vi "Read Log File Directory.vi"(8 "error in (no error)":errorcluster, 11 "Check Size Message in":refnum<class "Check Size Message.lvclass">) -> (0 "error out":errorcluster, 2 "Log File Directory":string, 3 "Check Size Message out":refnum<class "Check Size Message.lvclass">)   [LabVIEW 2020, in "AIM ARINC 664 Engine.lvlib" / "Implementation.lvlib" / "Frame Logging.lvlib" / "Check Size Message.lvclass"]
uses:
  Check Size Message.lvclass
  Check Size Message.lvclass/Check Size Message.ctl
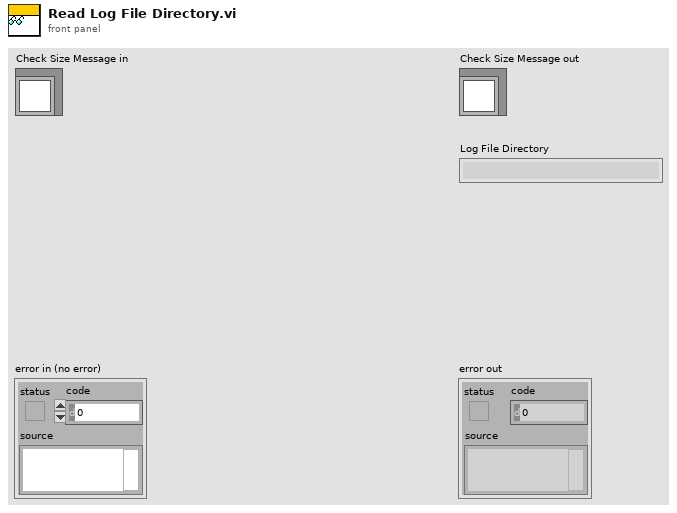
[diagram p1: front panel]
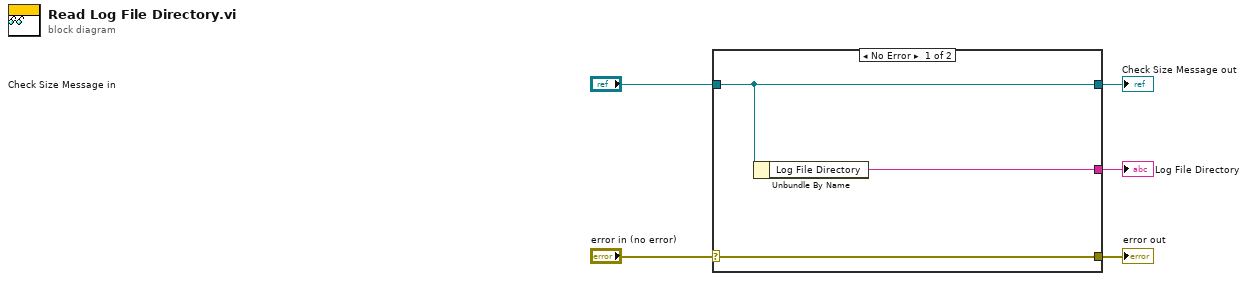
[diagram p0: block diagram]
diagram:
  n1 = case shown="No Error" "error in (no error)" {
    selector: "error in (no error)" -> [w8 w9]
    tunnel: [w8 w9] -> w4
    tunnel: [w7 w10] -> w2
    tunnel: "Check Size Message in" -> [w7 w10]
    tunnel: [w6 _] -> w1
    frame No Error {
      n2 = Unbundle By Name(w7) -> ("Log File Directory"=w6:string)
    }
    frame Error {
    }
  }
  "error out" <- w4
  "Check Size Message out" <- w2
  "Log File Directory" <- w1
